vi "format_plot.vi"(5 "Box Plot Width":dbl=10.0 format="%#_13g", 7 "Line Color":u32(colorbox)=16448250, 8 "error in (no error)":errorcluster, 10 "Number of Plots":i32, 11 "XY Graph":refnum<vi>) -> (0 "error out":errorcluster)   [LabVIEW 2021, in "statistics.lvlib"]
uses:
  statistics.lvlib
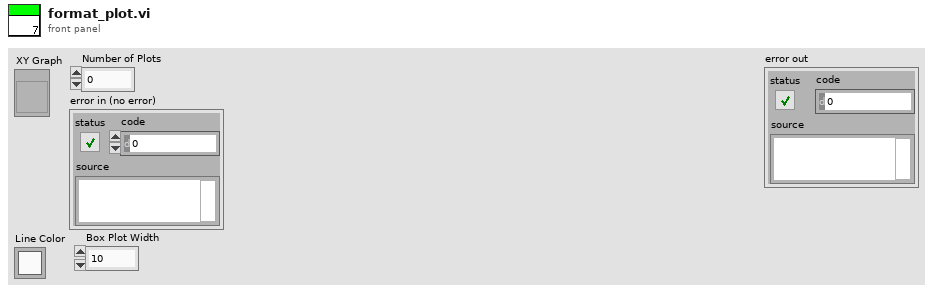
[diagram p1: front panel]
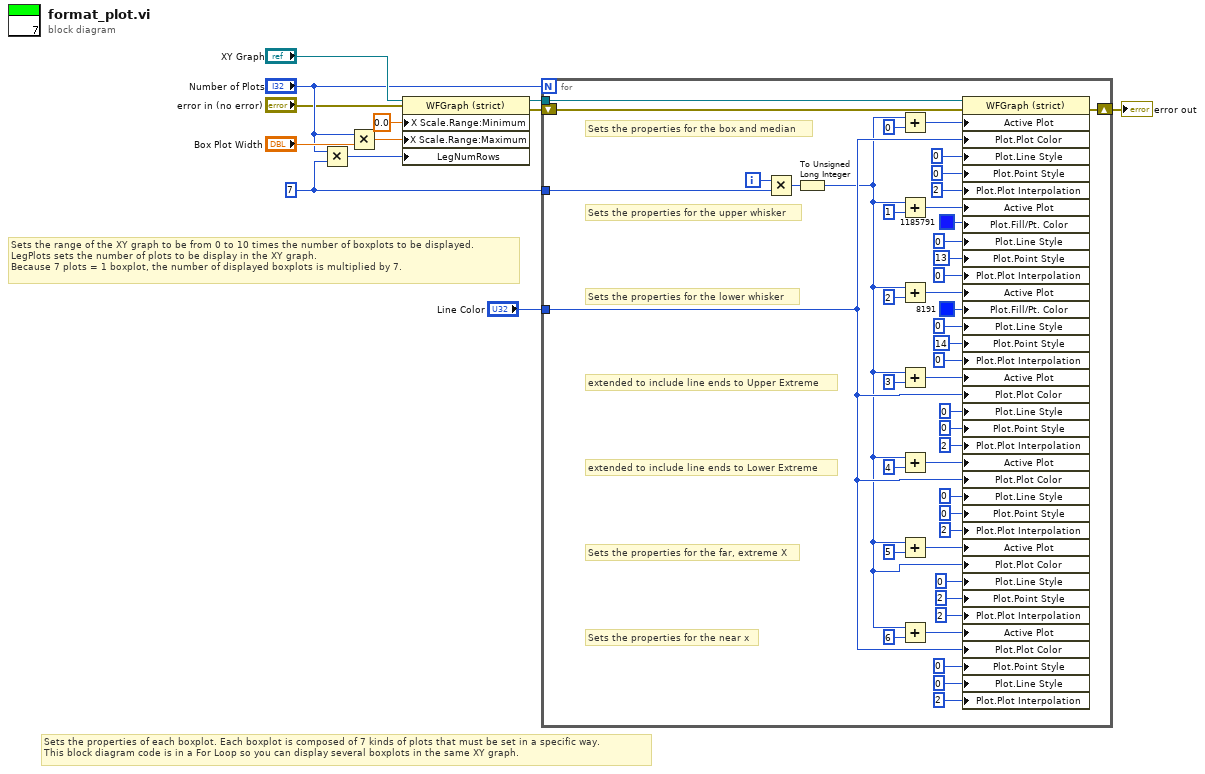
[diagram p0: block diagram]
diagram:
  w4 = 7 ("y")
  # "Sets the range of the XY graph to be from 0 to 10 times the number of boxplots to be displayed.  \nLegPlots sets the number of plots to be display in the XY graph. \nBecause 7 plots = 1 boxplot, the number of displayed boxplots is multiplied by 7."
  # "Sets the properties of each boxplot. Each boxplot is composed of 7 kinds of plots that must be set in a specific way. \nThis block diagram code is in a For Loop so you can display several boxplots in the same XY graph."
  n1 = Multiply(x="Number of Plots", y=w4) -> (x*y=w12:i32)
  n2 = Multiply(x="Number of Plots", y="Box Plot Width") -> (x*y=w9:dbl)
  n3 = property on="Property Node" class="WFGraph (strict)"(reference="XY Graph", error in="error in (no error)", "X Scale.Range:Minimum"=0.0 ("Legend:Plots Shown"), "X Scale.Range:Maximum"=w9, "LegNumRows"=w12) -> (reference out=w8:refnum<vi>, error out=w5:errorcluster)
  n4 = for {
    N: "Number of Plots" -> [_]
    tunnel: w8 -> [w57]
    shift-right: [w32] -> w3
    shift-left: w5 -> [w50]
    tunnel: w4 -> [w17]
    tunnel: "Line Color" -> [w14]
    i -> [w53]
    # "Sets the properties for the box and median"
    # "Sets the properties for the near x"
    # "Sets the properties for the far, extreme X"
    # "extended to include line ends to Upper Extreme"
    # "extended to include line ends to Lower Extreme"
    # "Sets the properties for the lower whisker"
    # "Sets the properties for the upper whisker"
    n5 = Multiply(x=w53, y=w17) -> (x*y=w26:i32)
    n6 = To Unsigned Long Integer(number=w26) -> (unsigned 32bit integer=w13:u32)
    n7 = Add(x=w13, y=u32 0) -> (x+y=w55:u32)
    n8 = Add(x=w13, y=u32 1) -> (x+y=w48:u32)
    n9 = Add(x=w13, y=u32 2) -> (x+y=w42:u32)
    n10 = Add(x=w13, y=u32 3) -> (x+y=w38:u32)
    n11 = Add(x=w13, y=u32 4) -> (x+y=w33:u32)
    n12 = Add(x=w13, y=u32 5) -> (x+y=w30:u32)
    n13 = Add(x=w13, y=u32 6) -> (x+y=w25:u32)
    n14 = property on="Property Node" class="WFGraph (strict)"(reference=w57, error in=w50, "Active Plot"=w55, "Plot.Plot Color"=w14, "Plot.Line Style"=u8 0, "Plot.Point Style"=u8 0, "Plot.Plot Interpolation"=u8 2, "Active Plot"=w48, "Plot.Fill/Pt. Color"=u32 1185791 ("Plot.Fill/Point Color"), "Plot.Line Style"=u8 0 ("Plot.Line Style 2"), "Plot.Point Style"=u8 13 ("Plot.Point Style 2"), "Plot.Plot Interpolation"=u8 0 ("Active Cursor"), "Active Plot"=w42, "Plot.Fill/Pt. Color"=u32 8191 ("Plot.Fill/Point Color"), "Plot.Line Style"=u8 0 ("Plot.Line Style 3"), "Plot.Point Style"=u8 14 ("Plot.Point Style 3"), "Plot.Plot Interpolation"=u8 0, "Active Plot"=w38, "Plot.Plot Color"=w14, "Plot.Line Style"=u8 0 ("Plot.Line Style 4"), "Plot.Point Style"=u8 0 ("Plot.Point Style 4"), "Plot.Plot Interpolation"=u8 2, "Active Plot"=w33, "Plot.Plot Color"=w14, "Plot.Line Style"=u8 0 ("Plot.Line Style 5"), "Plot.Point Style"=u8 0 ("Plot.Point Style 5"), "Plot.Plot Interpolation"=u8 2, "Active Plot"=w30, "Plot.Plot Color"=w13, "Plot.Line Style"=u8 0 ("Plot.Line Style 5"), "Plot.Point Style"=u8 2 ("Plot.Point Style 5"), "Plot.Plot Interpolation"=u8 2, "Active Plot"=w25, "Plot.Plot Color"=w14, "Plot.Point Style"=u8 0 ("Plot.Point Style 5"), "Plot.Line Style"=u8 0 ("Plot.Line Style 5"), "Plot.Plot Interpolation"=u8 2) -> (error out=w32:errorcluster)  [unwired: 1 out]
  }
  "error out" <- w3
